vi "Extrae_SetTemp.vi"(10 "String":string="Set Temperatura 4.2K at 20K/min, FastSettle") -> (1 "Array":string[](array[string]))   [LabVIEW 2017]
panel:
  # "Set Temperatura 4.2K at 20K/min, FastSettle, Wait"
  # "Set Temperatura 4.2K at 20K/min, FastSettle, Sweep&meas"
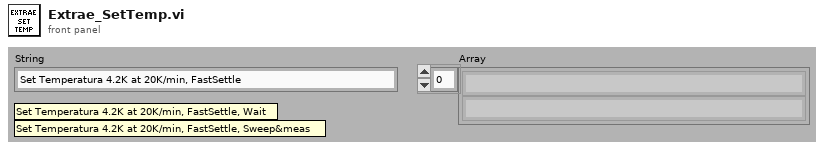
[diagram p1: front panel]
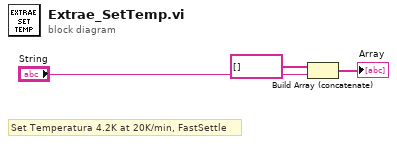
[diagram p0: block diagram]
diagram:
  # "Set Temperatura 4.2K at 20K/min, FastSettle"
  n1 = Build Array (concatenate)(string[] [] ("Array I"), "String") -> (→"Array":string[])
